vi "Process.vi"(8 "error in":errorcluster, 11 "SignalSenderLoop":refnum<class "SignalSenderLoop.lvclass">) -> (0 "error out":errorcluster, 3 "SignalSenderLoop out":refnum<class "SignalSenderLoop.lvclass">)   [LabVIEW 2020, in "SignalSenderLoop.lvclass"]
doc: "---------------------------------------------------------------\nJKI State Machine Objects™\nhttp://jki.net/state-machine-objects/\nCopyright (C) 2005-2015, JKI <info@jki.net>\nALL RIGHTS RESERVEDJKI State Machine Objects (SMO) 1.0.0.5\nJKI - JKI\nCopyright (c) 2016, JKI"
uses:
  SignalSenderLoop.lvclass
  C:/Program Files (x86)/National Instruments/LabVIEW 2020/vi.lib/JKI/JKI SMO/SMO/SMO.lvclass
  subvi/SignalFrameSet.ctl
  <vilib>/JKI/JKI SMO/SMO/Typedefs/Parent Call--Enum.ctl
  <vilib>/JKI/JKI SMO/SMO/SMO.lvclass/SMO.ctl
  <vilib>/Platform/TimedLoop/XDataNode/timing_clust.ctl
  <vilib>/Platform/TimedLoop/XDataNode/nitl_modes.ctl
  <vilib>/Platform/TimedLoop/XDataNode/wakeup.ctl
  <vilib>/JKI/JKI SMO/SMO/Private/ReftoDVR--SMO.vi
  <vilib>/xnet/xnet.llb/XNET Write (Signal Single-point).vi
  <vilib>/Utility/error.llb/Error Cluster From Error Code.vi
  <vilib>/Platform/TimedLoop/XDataNode/XDataNode.xnode
  <vilib>/ErrorRing/Error Ring.xnode
  <vilib>/JKI/JKI SMO/SMO/SMO.lvclass
  <vilib>/Platform/TimedLoop/XDataNode/XDNodeRunTimeDep.lvlib
panel:
  out "周期":i64
  out "SignalCommdExceptCounterChecksum":dbl[](array[numeric])=[60.0, 1.0] caption="data"
  out "SignalFrameSet":T1={"Port_No."="CAN1", "计数Count"=FALSE, "校验CheckSum"=FALSE, "MessageFrame"="ESP_1\nLRA110", "校验算法名称"=""}
  # "For instructions on how to use the JKI State Machine Objects, examples and video tutorials, visit:\nhttp://jki.net/state-machine-objects/\n\nJKI State Machine Objects™\nhttp://jki.net/state-machine-objects/\nCopyright (C) 2005-2015, JKI <info@jki.net>\nALL RIGHTS RESERVED"
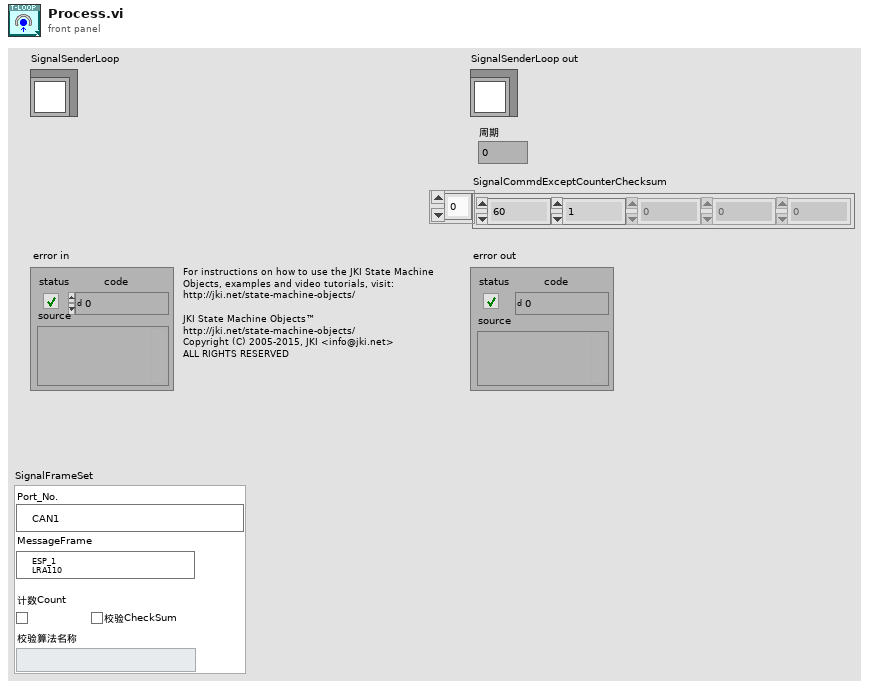
[diagram p1: front panel]
types:
  T1 = typedef "SignalSenderLoop.lvclass/SignalFrameSet.ctl" = cluster{"Port_No.":refnum<k21>, "计数Count":bool, "校验CheckSum":bool, "MessageFrame":refnum<k21>, "校验算法名称":string}
  T2 = typedef "SMO.lvclass/Parent Call--Enum.ctl" = enum16{"Allows parent to run", "Does not request parent to run"}
  T3 = typedef "XDNodeRunTimeDep.lvlib/timing_clust.ctl" = cluster{"Expected End [f-1]":u64, "Actual End [f-1]":u64, "Finished Late? [f-1]":bool, "Expected End [i-1]":u64, "Actual End [i-1]":u64, "Finished Late? [i-1]":bool, "Expected Start [i]":u64, "Actual Start [i]":u64, "Expected Start [f]":u64, "Actual Start [f]":u64, "Source Name":string, "Structure Name":string, "Period":i64, "Deadline":i64, "Offset":i64, "Start":i64, "Priority":i32, "Timeout":i32, "Mode":T4, "Wakeup Reason":T5, "Error":errorcluster, "Source Type":string, "Secondary Source Type":string, "Global End Time":u64, "Global Start Time":u64, "Frame Duration":u64, "Iteration Duration":u64, "Assigned CPU":i32, "I/O Scan Engine Mode":u32}
  T4 = typedef "XDNodeRunTimeDep.lvlib/nitl_modes.ctl" = enum32{"No Change", "Process missed periods, maintain original phase", "Discard missed periods, maintain original phase", "Process missed periods, ignore original phase", "Discard missed periods, ignore original phase"}
  T5 = typedef "XDNodeRunTimeDep.lvlib/wakeup.ctl" = enum32{"Normal", "Aborted", "Asynchronous wakeup", "Timing source error", "Timed loop error", "Timeout"}
  T6 = typedef "SignalSenderLoop.lvclass/PrivateEvents--Cluster.ctl" = cluster{"AsyncMethod":refnum<user-event>, "SignalCMDArry":refnum<user-event>}
  T7 = typedef "SMO.lvclass/Protected Events.ctl" = cluster{"StopProcesses":refnum<user-event>, "AbortProcesses":refnum<user-event>, "Config Changed":refnum<user-event>, "Dependency":refnum<user-event>}
  T8 = typedef "SignalSenderLoop.lvclass/PrivateEvents--SignalSenderLoop.SignalCMDArry.ctl" = dbl[]
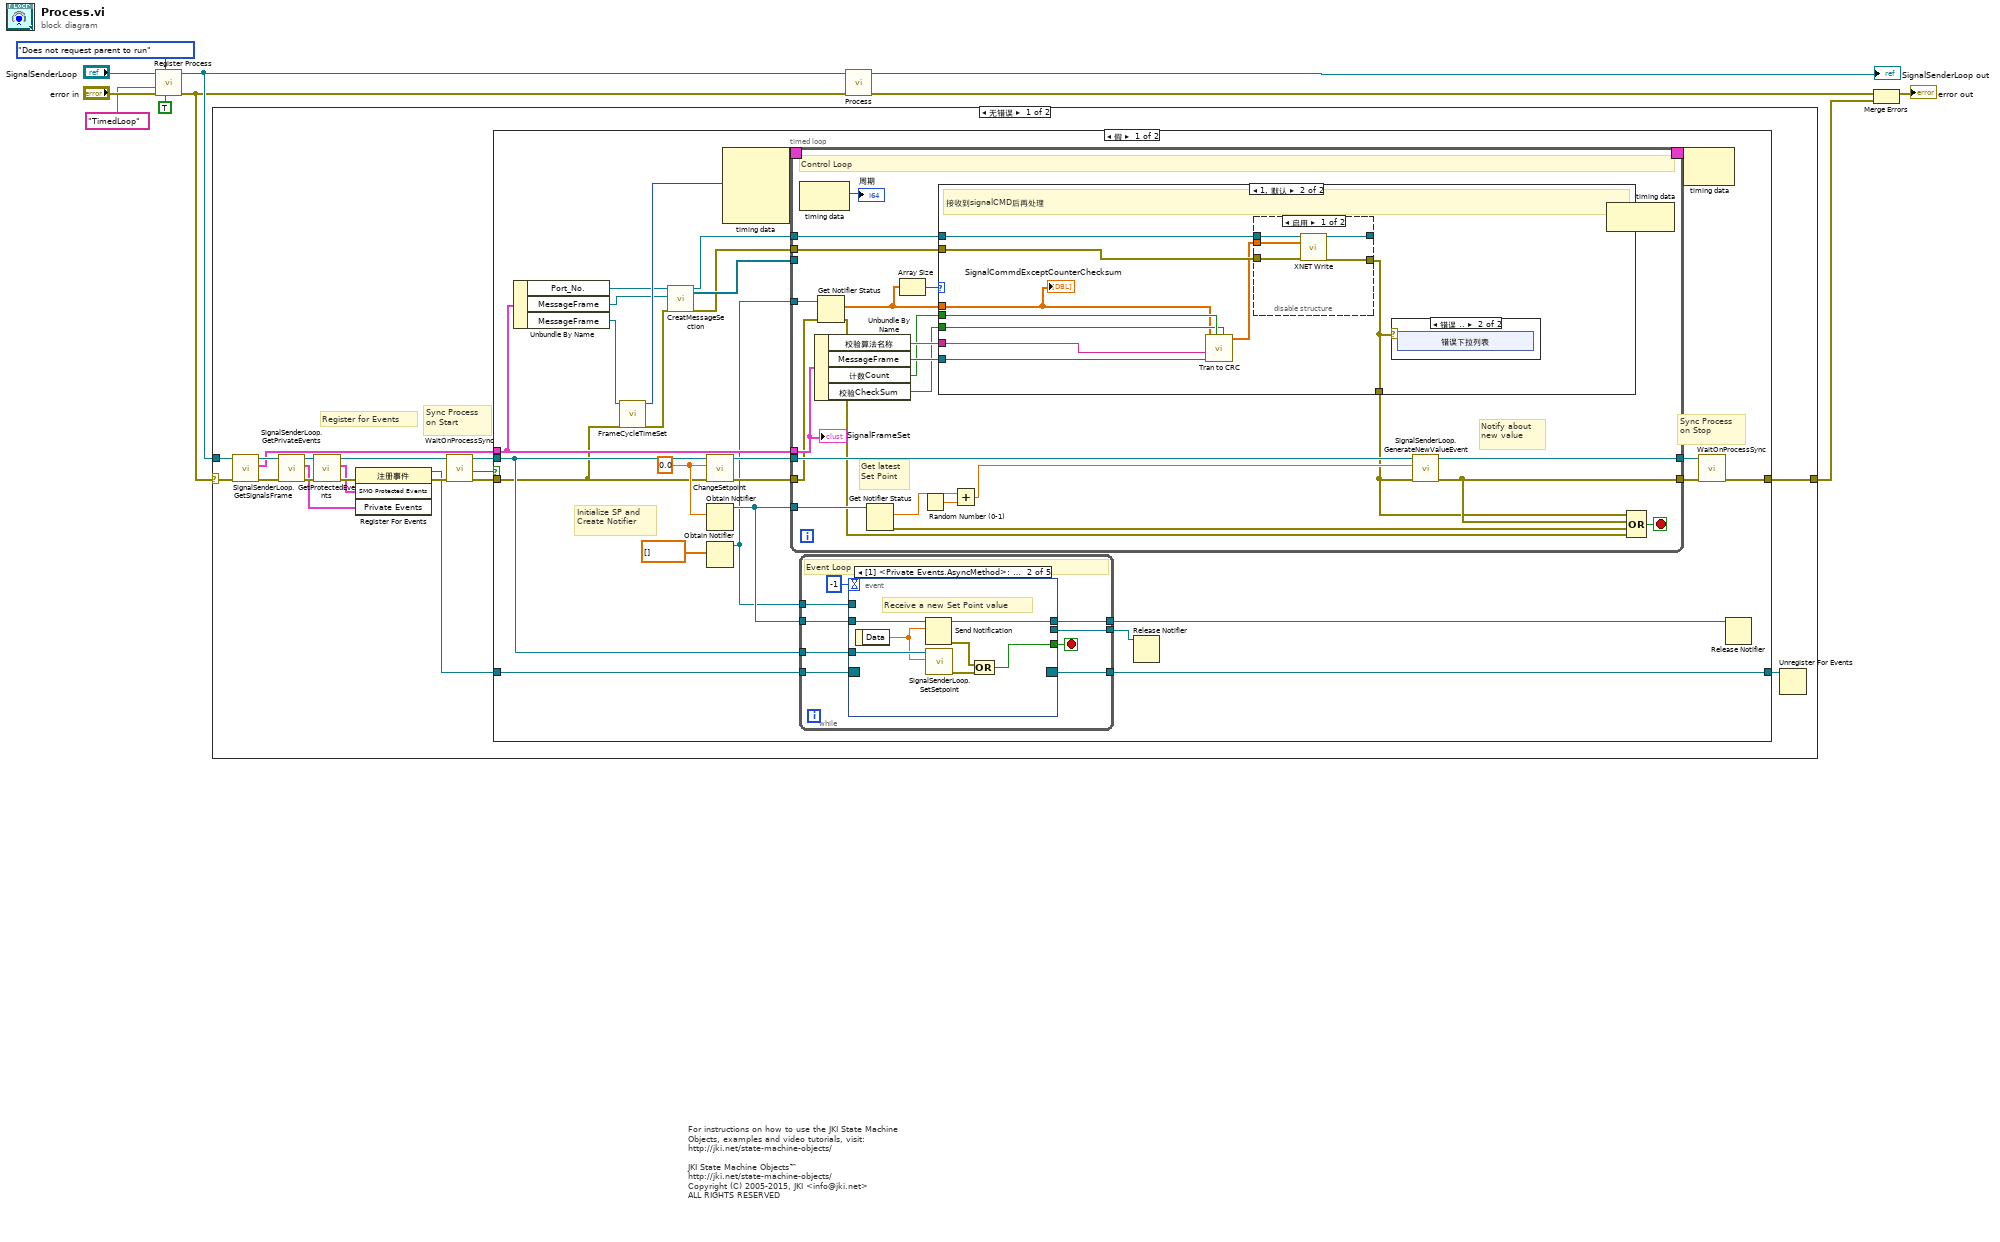
[diagram p0: block diagram]
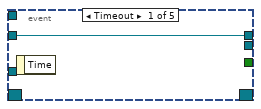
[diagram p2: hidden frame]
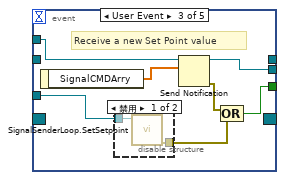
[diagram p3: hidden frame]
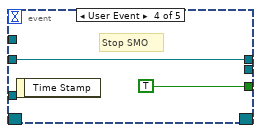
[diagram p5: hidden frame]
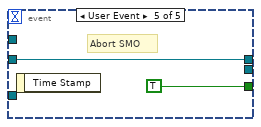
[diagram p6: hidden frame]
diagram:
  # "For instructions on how to use the JKI State Machine Objects, examples and video tutorials, visit:\nhttp://jki.net/state-machine-objects/\n\nJKI State Machine Objects™\nhttp://jki.net/state-machine-objects/\nCopyright (C) 2005-2015, JKI <info@jki.net>\nALL RIGHTS RESERVED"
  n1 = call <vilib>:"Register Process.vi"("Forces Self to Run (F)"=TRUE, "Parent Call"=Parent_Call--Enum."Does not request parent to run", "error in (no error)"="error in", "Process Name (optional)"="TimedLoop", "SMO"="SignalSenderLoop") -> ("error out"=w1:errorcluster, "SMO out"=w2:refnum<class "SignalSenderLoop.lvclass">)  [unwired: 5 in]
  n2 = case shown="无错误" w1 {
    selector: w1 -> [w15 w138]
    tunnel: w2 -> [w16 _]
    tunnel: [w21 w138] -> w6
    frame No Error {
      # "Sync Process\non Start"
      # "Register for Events"
      n3 = call "SignalSenderLoop.GetSignalsFrame.vi"("error in (no error)"=w15, "SignalSenderLoop"=w16) -> ("error out"=w12:errorcluster, "SignalFrameSet"=w13:T1, "SignalSenderLoop out"=w14:refnum<class "SignalSenderLoop.lvclass">)  [unwired: 7 in]
      n4 = call "SignalSenderLoop.GetPrivateEvents.vi"("error in (no error)"=w12, "SignalSenderLoop"=w14) -> ("error out"=w18:errorcluster, "Private Events"=w17:T6, "SignalSenderLoop out"=w19:refnum<class "SignalSenderLoop.lvclass">)  [unwired: 7 in]
      n5 = call <vilib>:"GetProtectedEvents.vi"("error in (no error)"=w18, "SMO"=w19) -> ("error out"=w24:errorcluster, "SMO Protected Events"=w23:T7, "SMO out"=w25:refnum<class "SignalSenderLoop.lvclass">)  [unwired: 7 in]
      n6 = register-events(error in=w24, w23, w17) -> (reference out=w22:refnum<event-registration>, error out=w26:errorcluster)  [unwired: 1 in]
      n7 = call <vilib>:"WaitOnProcessSync.vi"("error in (no error)"=w26, "SMO"=w25) -> ("error out"=w28:errorcluster, "Don't run?"=w29:bool, "SMO out"=w27:refnum<class "SignalSenderLoop.lvclass">)  [unwired: 7 in]
      n8 = case shown="假" w29 {
        tunnel: w28 -> [w32 w136]
        tunnel: w27 -> [w43 _]
        tunnel: w22 -> [w50 w137]
        tunnel: [w51 w136] -> w21
        tunnel: [w49 w137] -> w20
        tunnel: w13 -> [w42 _]
        frame False {
          w45 = 0.0 ("Setpoint")
          # "Initialize SP and\nCreate Notifier"
          # "Sync Process\non Stop"
          n9 = Unbundle By Name(w42) -> ("Port_No."=w35:refnum<k21>, "MessageFrame"=w34:refnum<k21>, "MessageFrame"=w41:refnum<k21>)
          n10 = call "FrameCycleTimeSet.vi"("XNET Frame"=w41, "error in (no error)"=w32) -> ("MessageFrameCycleTime"=w37:i32, "错误输出"=w31:errorcluster)  [unwired: 15 in, 1 out]
          n11 = call "CreatMessageSection.vi"("Port_No."=w35, "MessageFrame"=w34, "错误输入（无错误）"=w31) -> ("session out"=w33:refnum<k21>, "Sigs"=w36:refnum<k21>[], "error out"=w30:errorcluster)  [unwired: 14 in]
          n12 = call "ChangeSetpoint.vi"("error in (no error)"=w32, "Setpoint"=w45, "SignalSenderLoop"=w43) -> ("error out"=w47:errorcluster, "SignalSenderLoop out"=w46:refnum<class "SignalSenderLoop.lvclass">)  [unwired: 7 in]
          n13 = Obtain Notifier(notification data type=w45) -> (notifier out=w44:refnum<notifier>)  [unwired: 3 in, 2 out]
          n14 = Obtain Notifier(notification data type=dbl[] []) -> (notifier out=w38:refnum<notifier>)  [unwired: 3 in, 2 out]
          n15 = node-c288(w37) -> (w55:T3)  [unwired: 3 in]
          n16 = timed-loop {
            timing: w55 -> [_]
            timing-out: [_] -> w54
            tunnel: w46 -> [w100]
            tunnel: w47 -> [w88]
            tunnel: w44 -> [w108]
            tunnel: [w105] -> w53
            tunnel: [w104] -> w52
            tunnel: w42 -> [w99]
            tunnel: w38 -> [w96]
            tunnel: w36 -> [_]
            tunnel: w33 -> [w89]
            tunnel: w30 -> [w87]
            stop <- w106 stop-if-true
            # "Notify about\nnew value"
            # "Get latest\nSet Point"
            # "Control Loop"
            n17 = node-c288() -> (→"周期":i64)  [unwired: 1 in]
            n18 = Unbundle By Name(w99) -> ("校验算法名称"=w98:string, "MessageFrame"=w97:refnum<k21>, "计数Count"=w92:bool, "校验CheckSum"=w91:bool)
            n19 = Get Notifier Status(notifier=w96, error in (no error)=w88) -> (current notification=w94:dbl[], error out=w95:errorcluster)  [unwired: 3 out]
            n20 = Get Notifier Status(notifier=w108) -> (current notification=w101:dbl, error out=w107:errorcluster)  [unwired: 1 in, 3 out]
            n21 = Array Size(array=w94) -> (size(s)=w93:i32)
            n22 = Random Number (0-1)() -> (number: 0 to 1=w103:dbl)
            n23 = case shown="1, 默认" w93 {
              tunnel: w89 -> [_ w109]
              tunnel: w87 -> [_ w117]
              tunnel: w98 -> [_ w116]
              tunnel: w97 -> [_ w115]
              tunnel: w94 -> [_ w112]
              tunnel: w92 -> [_ w114]
              tunnel: w91 -> [_ w113]
              tunnel: [_ w110] -> w86
              frame 0 {
                # "没收到signalCMD不发送任何报文"
              }
              frame 1, Default {
                # "接收到signalCMD后再处理"
                n24 = call "Tran to CRC.vi"("CheckSum？"=w113, "Count"=w114, "MessageFrame"=w115, "校验算法名称"=w116, "CAN_commd"=w112) -> ("SignalsArryOut"=w111:dbl[])  [unwired: 4 in, 2 out]
                n25 = disable-structure shown="启用" {
                  disable-tunnel: w111 -> [w127 _]
                  disable-tunnel: w117 -> [w126 w128]
                  disable-tunnel: [w125 w128] -> w110
                  disable-tunnel: w109 -> [w124 _]
                  disable-tunnel: [w123 _] -> _
                  frame Enabled {
                    n26 = call-poly <vilib>:"XNET Write.vi"("session in"=w124, "data"=w127, "error in (no error)"=w126) -> ("session out"=w123:refnum<k21>, "error out"=w125:errorcluster)  [unwired: 11 out]
                  }
                  frame Disabled {
                  }
                }
                n27 = case shown="错误 .." w110 {
                  frame No Error {
                  }
                  frame Error {
                    n28 = xnode "错误下拉列表"() -> ()  [unwired: 1 out]
                  }
                }
                "SignalCommdExceptCounterChecksum" <- w112
              }
            }
            n29 = Add(x=w101, y=w103) -> (x+y=w102:dbl)
            n30 = call "SignalSenderLoop.GenerateNewValueEvent.vi"("error in (no error)"=w86, "New Value"=w102, "SignalSenderLoop"=w100) -> ("error out"=w104:errorcluster, "SignalSenderLoop out"=w105:refnum<class "SignalSenderLoop.lvclass">)  [unwired: 7 in]
            n31 = node-c288() -> ()  [unwired: 1 in, 1 out]
            n32 = Compound Arithmetic op=OR(w86, w104, w107, w95) -> (w106:bool)
            "SignalFrameSet" <- w99
          }
          n33 = while {
            tunnel: w50 -> [w63]
            tunnel: [w62] -> w49
            tunnel: [w59] -> w48
            tunnel: w44 -> [w60]
            tunnel: w43 -> [w58]
            tunnel: w38 -> [w57]
            tunnel: [w56] -> w39
            stop <- w61 stop-if-true
            # "Event Loop"
            n34 = event shown="[1] <Private Events.AsyncMethod>: 用户事件" {
              selector: w63 -> [_ _ _ _ _]
              dyn-events: [_ _ _ _ _] -> w62
              timeout: -1 -> [_ _ _ _ _]
              tunnel: [_ w66 w75 TRUE TRUE] -> w61
              tunnel: w60 -> [w65 w72 _ w82 w84]
              tunnel: [w65 w71 _ w82 w84] -> w59
              tunnel: w58 -> [_ w70 w79 _ _]
              tunnel: w57 -> [_ _ w74 _ _]
              tunnel: [_ _ w73 _ _] -> w56
              event Timeout {
                n35 = event-data() -> ()  [unwired: 1 in, 1 out]
              }
              event User Event {
                # "Receive a new Set Point value"
                n36 = event-data() -> ("Data"=w69:dbl)  [unwired: 1 in]
                n37 = Send Notification(notification=w69, notifier=w72) -> (notifier out=w71:refnum<notifier>, error out=w67:errorcluster)  [unwired: 1 in]
                n38 = call "SignalSenderLoop.SetSetpoint.vi"("Setpoint"=w69, "SignalSenderLoop"=w70) -> ("error out"=w68:errorcluster)  [unwired: 8 in, 1 out]
                n39 = Compound Arithmetic op=OR(w67, w68) -> (w66:bool)
              }
              event User Event {
                # "Receive a new Set Point value"
                n40 = event-data() -> ("SignalCMDArry"=w78:T8)  [unwired: 1 in]
                n41 = disable-structure shown="禁用" {
                  disable-tunnel: w79 -> [w81 _]
                  disable-tunnel: [w80 _] -> w77
                  frame Disabled {
                    n42 = call "SignalSenderLoop.SetSetpoint.vi"("SignalSenderLoop"=w81) -> ("error out"=w80:errorcluster)  [unwired: 9 in, 1 out]
                  }
                  frame Enabled {
                  }
                }
                n43 = Send Notification(notification=w78, notifier=w74) -> (notifier out=w73:refnum<notifier>, error out=w76:errorcluster)  [unwired: 1 in]
                n44 = Compound Arithmetic op=OR(w76, w77) -> (w75:bool)
              }
              event User Event {
                # "Stop SMO"
                n45 = event-data() -> ()  [unwired: 1 in, 1 out]
              }
              event User Event {
                # "Abort SMO"
                n46 = event-data() -> ()  [unwired: 1 in, 1 out]
              }
            }
          }
          n47 = Release Notifier(notifier=w39) -> ()  [unwired: 2 in, 3 out]
          n48 = node-c288(w54) -> ()  [unwired: 1 out]
          n49 = call <vilib>:"WaitOnProcessSync.vi"("error in (no error)"=w52, "SMO"=w53) -> ("error out"=w51:errorcluster)  [unwired: 7 in, 2 out]
          n50 = Release Notifier(notifier=w48) -> ()  [unwired: 2 in, 3 out]
        }
        frame True {
        }
      }
      n51 = Unregister For Events(event registration refnum=w20) -> ()  [unwired: 1 in, 1 out]
    }
    frame Error {
    }
  }
  n52 = call-parent "Process.vi"("error in"=w1, "SMO"=w2) -> ("error out"=w7:errorcluster, "SMO out"=→"SignalSenderLoop out":refnum<class "SignalSenderLoop.lvclass">)  [unwired: 8 in]
  n53 = Merge Errors(w7, w6) -> (→"error out":errorcluster)
